vi "FileExplorer.vi"(0 "FolderPath":path, 1 "Copy Button":bool, 2 "Expand/Collapse":bool, 5 "Tree":string[](tree), 7 "SearchBar":string, 11 "error in (no error)":errorcluster) -> (4 "Report":string, 15 "error out":errorcluster)   [LabVIEW 2021]
doc: "This Vi acts as a file explorer. It populates the subfolders and files present in the selected folder path in tree along with the data of Last Modified,Type and Size of files."
uses:
  Controls/Operations.ctl
  Controls/Data Cluster.ctl
  Controls/State.ctl
panel:
  # "Instructions:\n\n-> Select the folder path to populate the subfolders and files present in tree.\n-> A report is generated for the folders whose checkbox is selected in tree.\n-> Press Collapse All button to collapse all nodes in tree and Expand All to expand\n      all nodes in tree.\n->  Enter a folder name in search bar and click enter to expand the nodes of searched folder.\n-> Click column headers such as Last Modified to sort the column itemns in ascending \n      and descending order.\n-> Select file to copy and click Copy button which opens a dialog box to choose the\n      folder path where the files are copied."
  # "Instructions:\n\n-> Select the Folder Path to populate the subfolders and files present in it in tree.\n->  Can select multiple files of same folder and press Copy button to copy those files.\n->  Clicking a Copy button opens a dialog box to choose the destination folder path \n       where the files are copied.\n->  A report is generated for the folders whose checkbox is selected in tree.\n->  Press Collapse All button to collapse all nodes in tree and Expand all to expand \n       all nodes in tree.\n->   Enter a folder name in SearchBar and press Search to search for a particular folder\n       in tree.\n->   Press column headers such as Last Modified to sort the column items in ascending \n        or descending order."
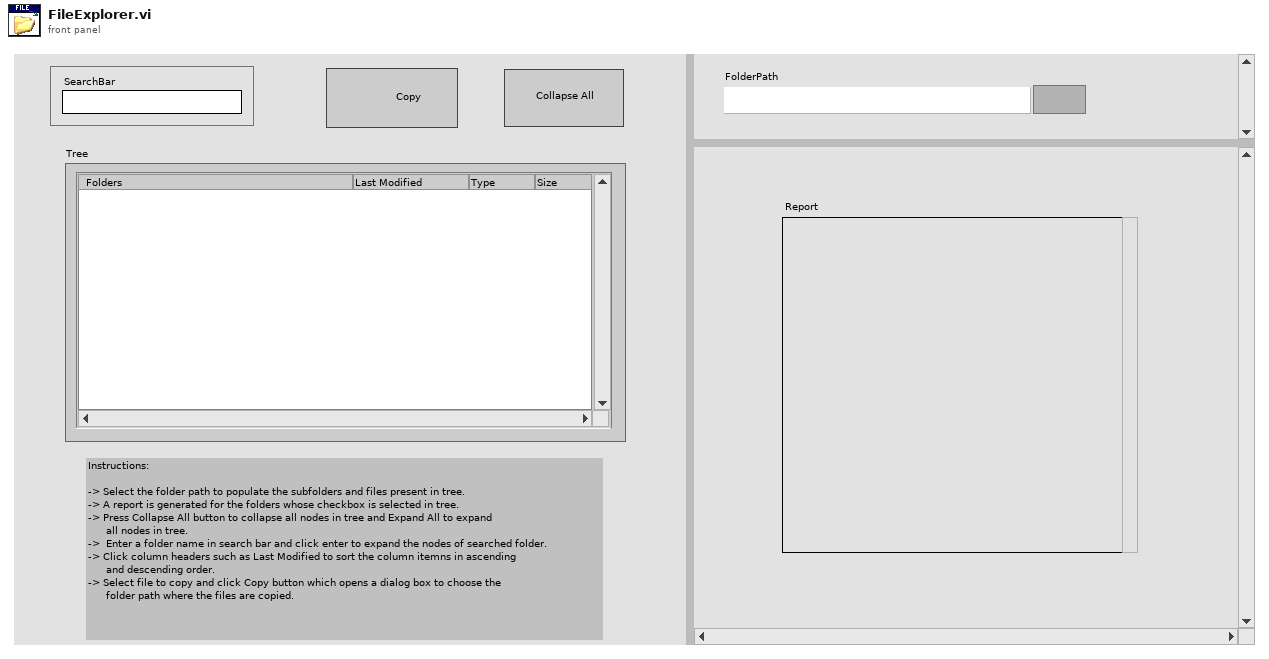
[diagram p1: front panel]
types:
  T1 = typedef "State.ctl" = cluster{"State":string, "Data":variant}
  T2 = typedef "Data Cluster.ctl" = cluster{"Stop user event":refnum<user-event>, "FolderPath":path, "FolderName":string, "FolderPathArray":path[], "FilePathArray":path[], "Index":i32, "No.of Folders":i32, "SelectedTags":string[], "SelectedFilePaths":path[], "SearchTag":string, "Column":i32, "Toggle":bool, "FolderTag":string, "ActiveTag":string, "ListBox":i32, "Report":string}
  T3 = typedef "Operations.ctl" = enum16{"Create", "Enqueue", "Enqueue N", "Enstack", "Dequeue", "Flush", "Release"}
  T4 = typedef "LVPoint32TypeDef.ctl" = cluster{"Horizontal":i32, "Vertical":i32}
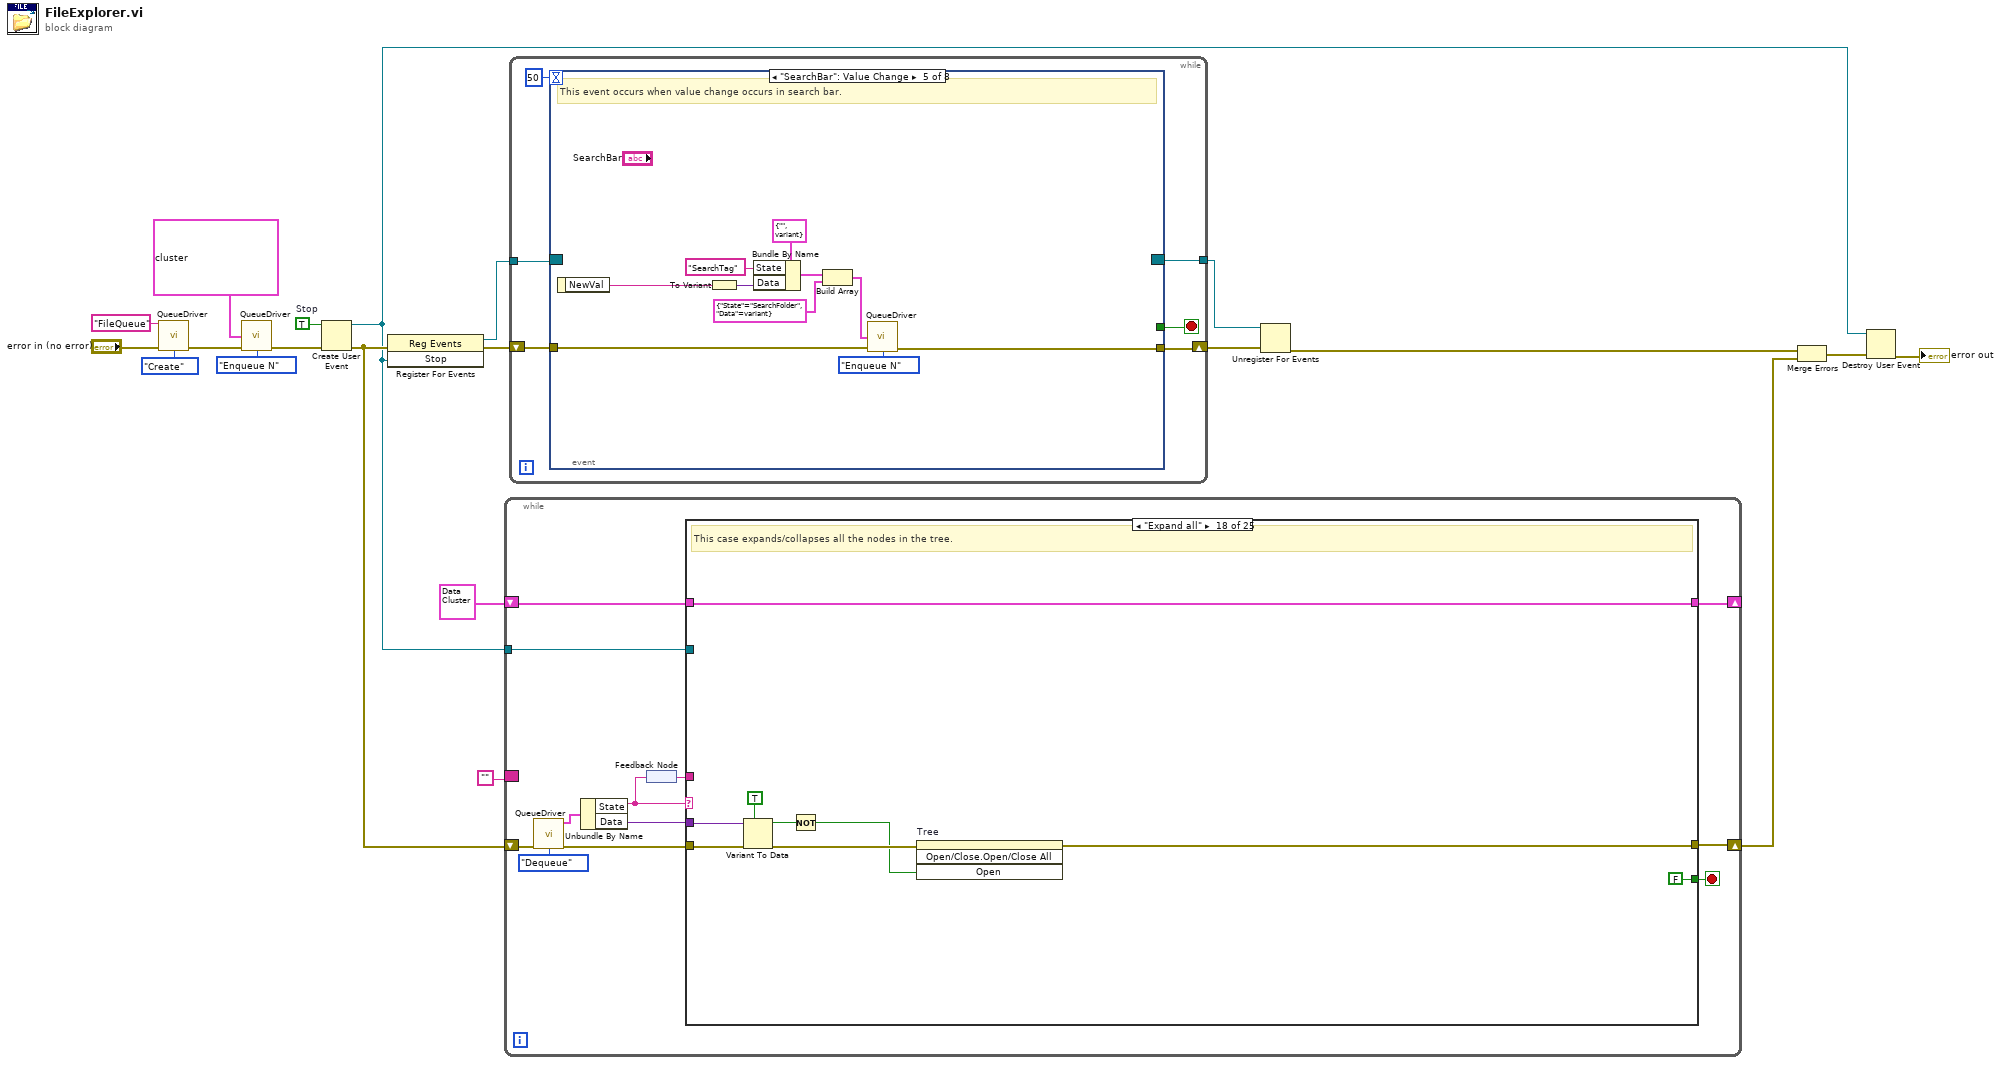
[diagram p0: block diagram]
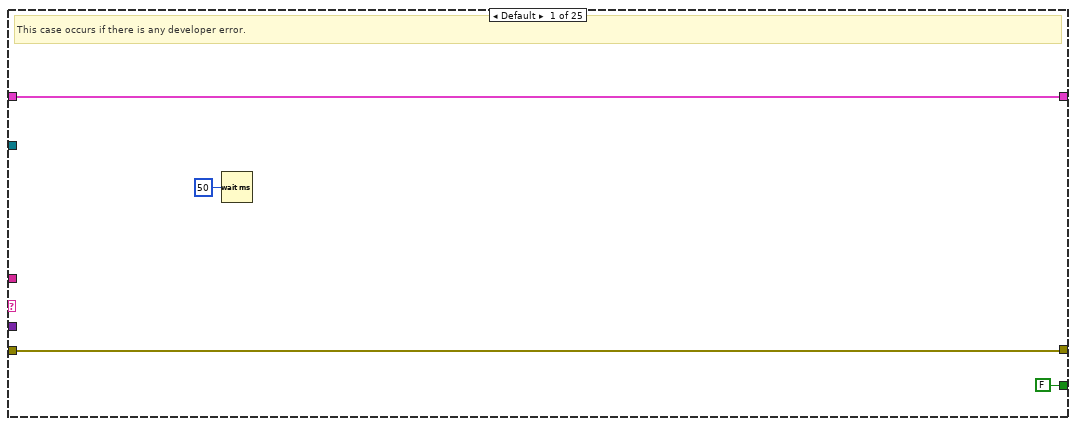
[diagram p2: hidden frame]
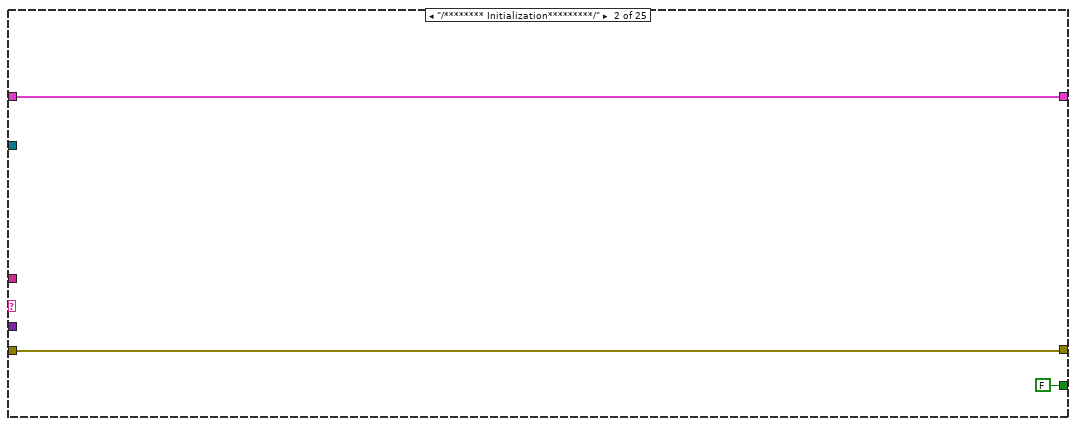
[diagram p3: hidden frame]
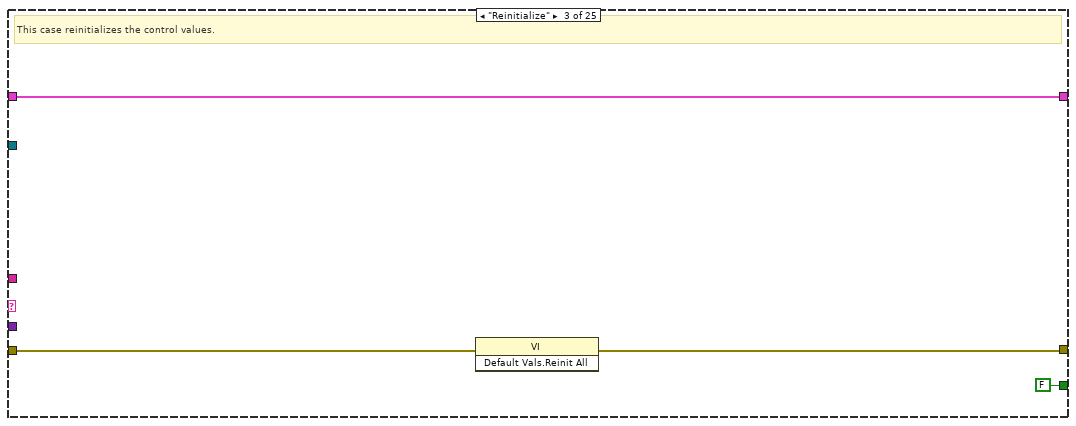
[diagram p4: hidden frame]
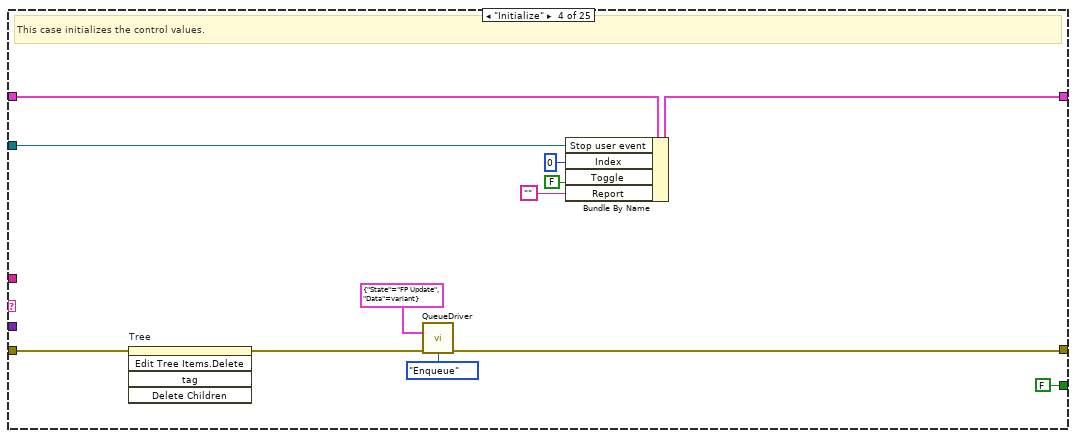
[diagram p5: hidden frame]
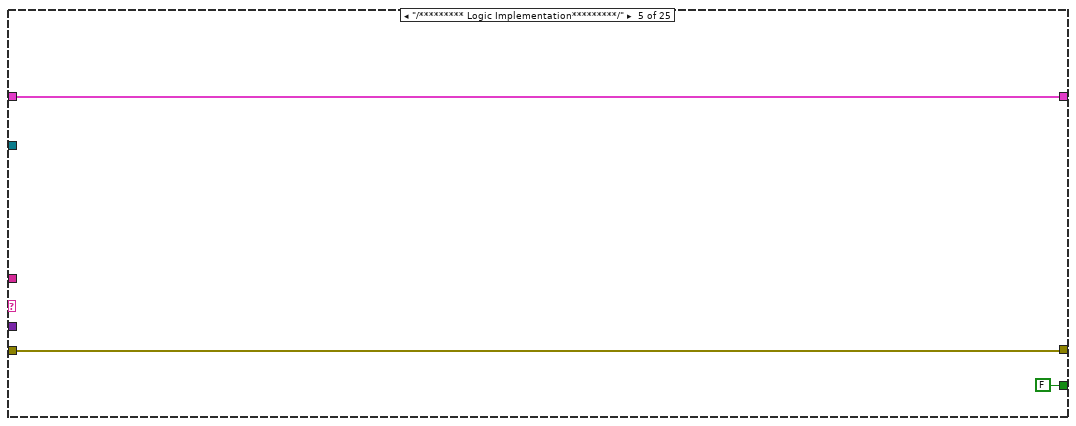
[diagram p6: hidden frame]
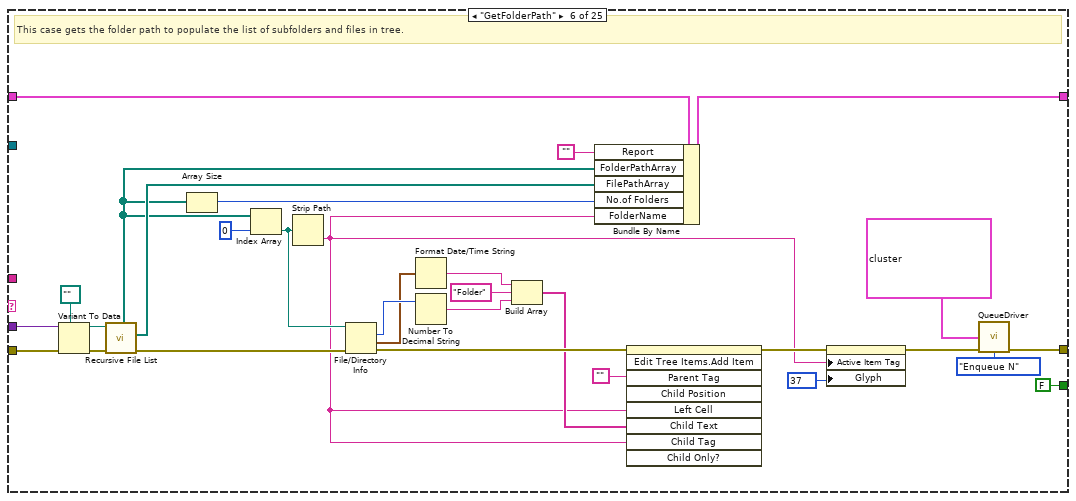
[diagram p7: hidden frame]
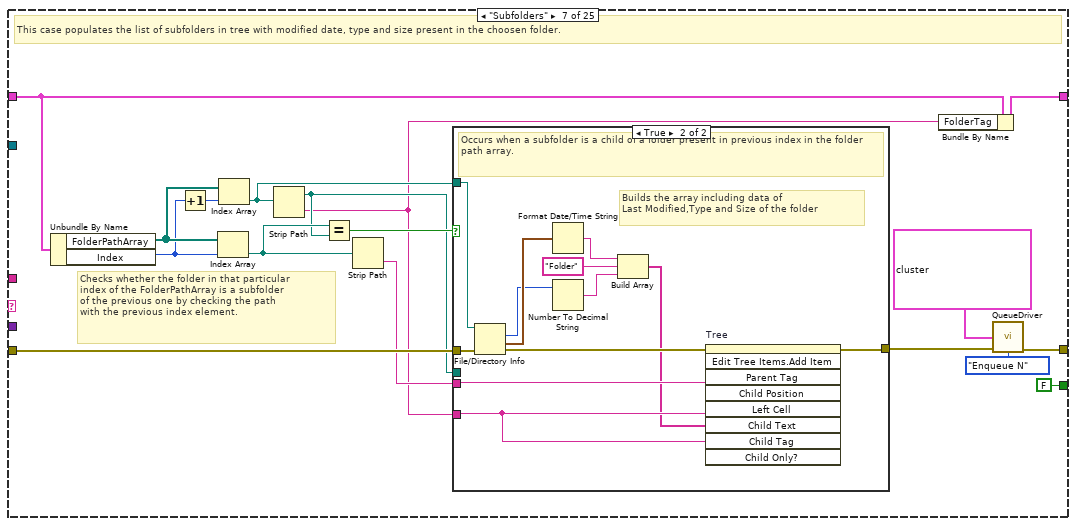
[diagram p8: hidden frame]
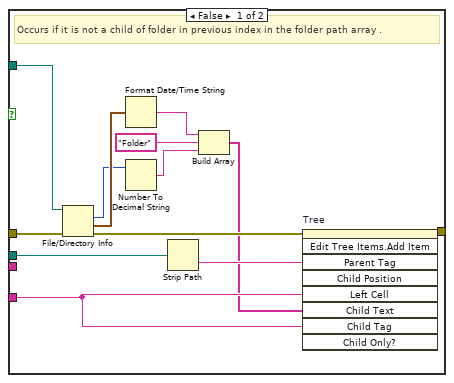
[diagram p9: hidden frame]
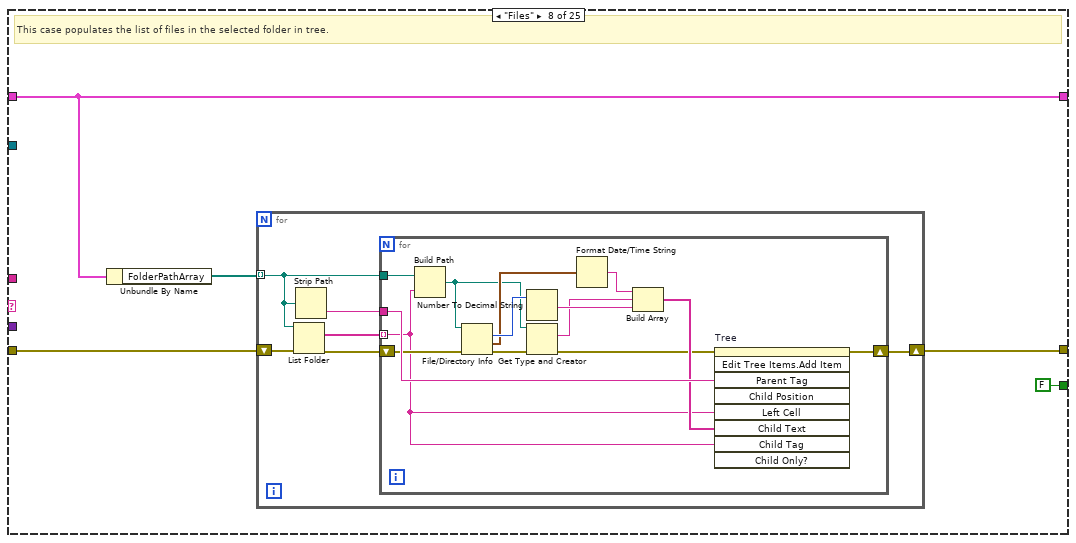
[diagram p10: hidden frame]
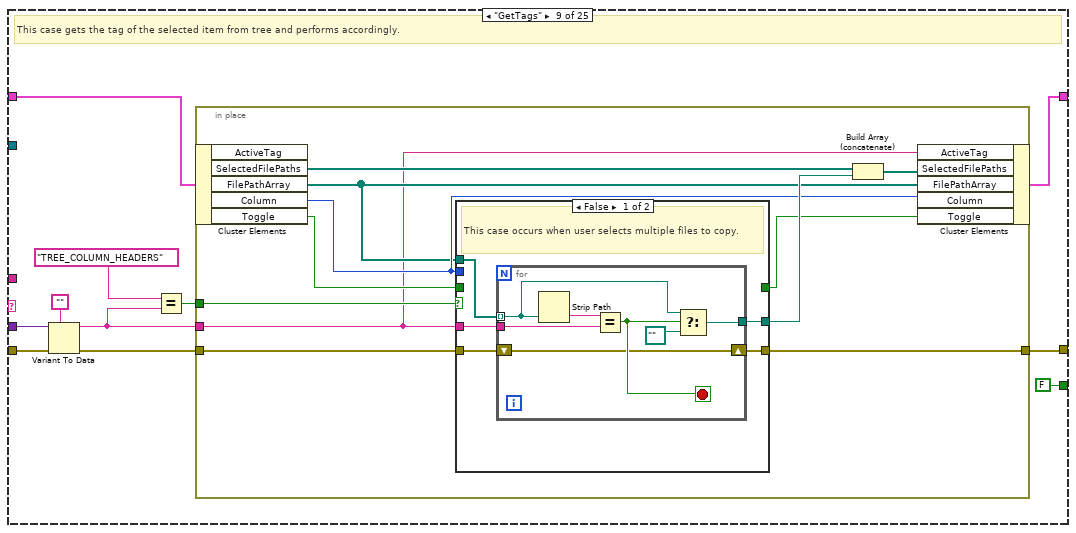
[diagram p11: hidden frame]
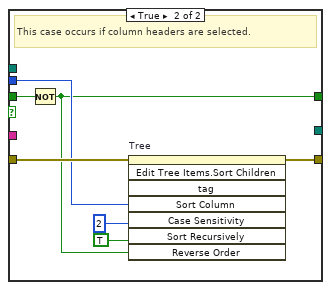
[diagram p12: hidden frame]
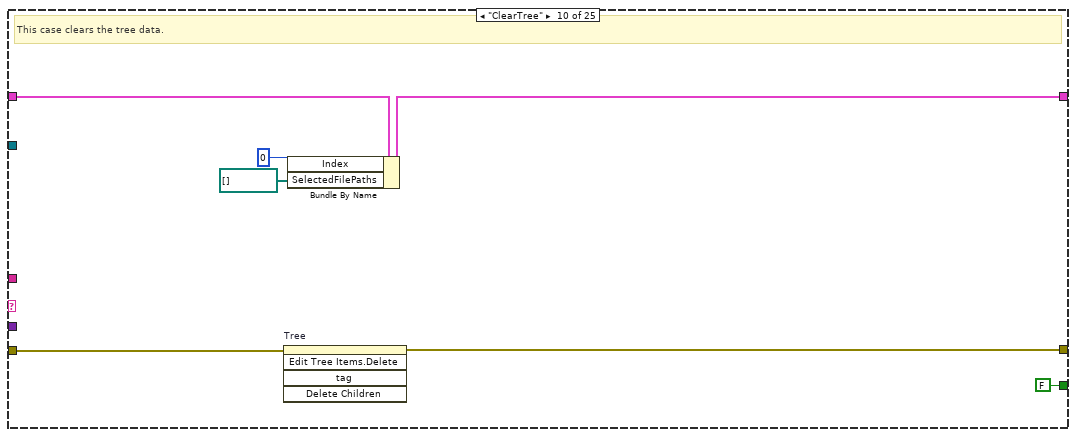
[diagram p13: hidden frame]
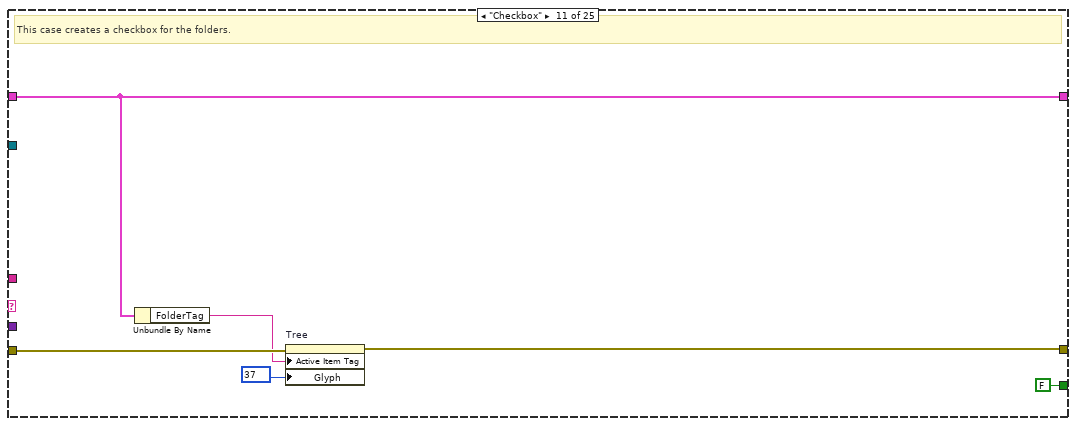
[diagram p14: hidden frame]
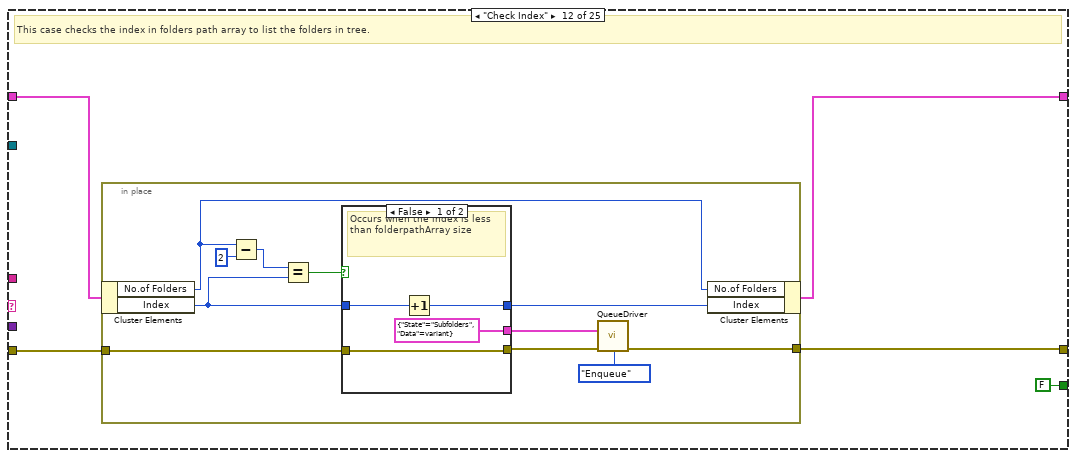
[diagram p15: hidden frame]
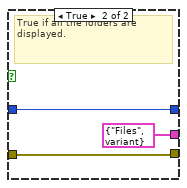
[diagram p16: hidden frame]
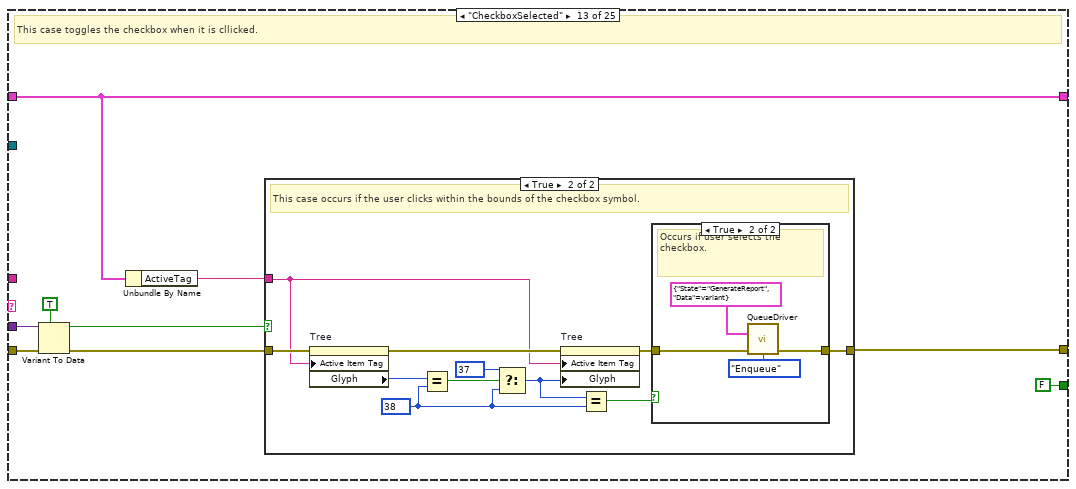
[diagram p17: hidden frame]
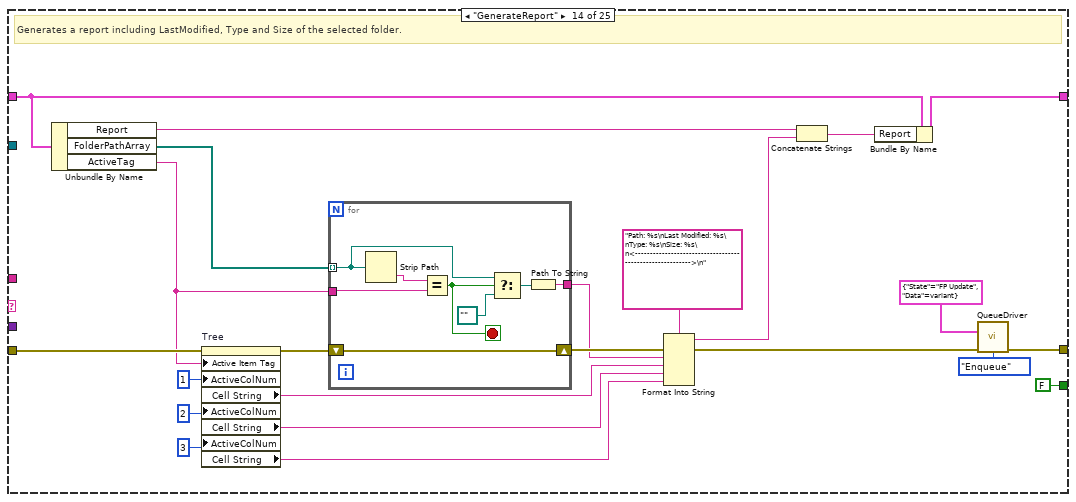
[diagram p20: hidden frame]
diagram:
  w20 = TRUE  # Stop
  n1 = call "QueueDriver.vi"("Queue Name"="FileQueue", "error in (no error)"="error in (no error)", "Operations"=Operations."Create") -> ("error out"=w15:errorcluster)  [unwired: 11 in, 1 out]
  n2 = call "QueueDriver.vi"("State[]"=T1[] [{"State"="Reinitialize", "Data"=variant}, {"State"="Initialize", "Data"=variant}], "error in (no error)"=w15, "Operations"=Operations."Enqueue N") -> ("error out"=w14:errorcluster)  [unwired: 11 in, 1 out]
  n3 = Create User Event(user event datatype=w20, error in=w14) -> (user event=w4:refnum<user-event>, error out=w17:errorcluster)
  n4 = register-events(error in=w17, w4) -> (reference out=w18:refnum<event-registration>, error out=w19:errorcluster)  [unwired: 1 in]
  n5 = while {
    shift-right: [w29] -> w6
    shift-left: w17 -> [w27]
    border: "" ("Empty String Constant") -> [_]
    tunnel: w4 -> [w23]
    shift-right: [w21] -> _
    shift-left: T2 {"Stop user event"=refnum, "FolderPath"=path "", "FolderName"="", "FolderPathArray"=[], "FilePathArray"=[], "Index"=0, "No.of Folders"=0, "SelectedTags"=[], "SelectedFilePaths"=[], "SearchTag"="", "Column"=0, "Toggle"=FALSE, "FolderTag"="", "ActiveTag"="", "ListBox"=0, "Report"=""} -> [w22]
    stop <- w28 stop-if-true
    n6 = call "QueueDriver.vi"("error in (no error)"=w27, "Operations"=Operations."Dequeue") -> ("Dequeued Element"=w25:T1, "error out"=w26:errorcluster)  [unwired: 12 in]
    n7 = Unbundle By Name(w25) -> ("State"=w32:string, "Data"=w30:variant)
    n8 = feedback-in #1(w32) -> ()
    n9 = feedback #1() -> (w31:string)
    n10 = case shown="\"Expand all\"" w32 {
      tunnel: w26 -> [w36 w39 w43 w52 w58 w88 w102 w134 w166 w202 w208 w214 w241 w281 w297 w303 w316 w337 w345 w348 w352 w355 w361 w381 w386]
      tunnel: w31 -> [_ _ _ _ _ _ _ _ _ _ _ _ _ _ _ _ _ _ _ _ _ _ w360 _ _]
      tunnel: w30 -> [_ _ _ _ _ w87 _ _ w165 _ _ _ w240 _ w296 _ _ w335 w343 _ _ _ _ _ _]
      tunnel: [w36 w39 w41 w46 w58 w79 w96 w132 w163 w203 w207 w213 w234 w262 w291 w299 w318 w332 w344 w348 w352 w355 w359 w381 w385] -> w29
      tunnel: [FALSE FALSE FALSE FALSE FALSE FALSE FALSE FALSE FALSE FALSE FALSE FALSE FALSE FALSE FALSE FALSE FALSE FALSE FALSE FALSE FALSE FALSE FALSE FALSE TRUE] -> w28
      tunnel: w23 -> [_ _ _ w54 _ _ _ _ _ _ _ _ _ _ _ _ _ _ _ _ _ _ _ _ _]
      tunnel: w22 -> [w35 w38 w42 w55 w57 w83 w92 w135 w158 w201 w209 w211 w238 w266 w294 w302 w313 w336 w341 w347 w351 w354 w358 w380 w382]
      tunnel: [w35 w38 w42 w53 w57 w82 w91 w135 w157 w200 w209 w210 w238 w265 w293 w302 w312 w336 w339 w347 w351 w354 w358 w380 w382] -> w21
      frame Default {
        # "This case occurs if there is any developer error."
        n11 = Wait (ms)(milliseconds to wait=u32 50) -> ()  [unwired: 1 out]
      }
      frame "/******** Initialization*********/" {
      }
      frame "Reinitialize" {
        # "This case reinitializes the control values."
        n12 = invoke on="Invoke Node" class="VI" method="Default Vals.Reinit All"(error in=w43) -> (error out=w41:errorcluster)  [unwired: 2 in, 2 out]
      }
      frame "Initialize" {
        # "This case initializes the control values."
        n13 = invoke on="Tree" class="Tree (strict)" method="Edit Tree Items.Delete"(error in=w52) -> (error out=w49:errorcluster)  [unwired: 4 in, 4 out]
        n14 = call "QueueDriver.vi"("State"=T1 {"State"="FP Update", "Data"=variant}, "error in (no error)"=w49, "Operations"=Operations."Enqueue") -> ("error out"=w46:errorcluster)  [unwired: 11 in, 1 out]
        n15 = Bundle By Name(cluster=w55, "Stop user event"=w54, "Index"=0, "Toggle"=FALSE, "Report"="" ("Empty String Constant")) -> (w53:T2)
      }
      frame "/********* Logic Implementation*********/" {
      }
      frame "GetFolderPath" {
        # "This case gets the folder path to populate the list of subfolders and files in tree."
        n16 = Variant To Data(error in=w88, type=path "" ("NewVal"), Variant=w87) -> (data=w84:path, error out=w85:errorcluster)
        n17 = call <vilib>:"Recursive File List.vi"("error in (no error)"=w85, "Folder Path"=w84) -> ("error out"=w72:errorcluster, "All Files in Dir"=w81:path[], "All Folders"=w77:path[])  [unwired: 5 in, 2 out]
        n18 = Array Size(array=w77) -> (size(s)=w76:i32)
        n19 = Index Array(array=w77, index=0) -> (element=w68:path)
        n20 = Strip Path(path=w68) -> (name=w64:string)  [unwired: 1 out]
        n21 = File/Directory Info(path=w68, error in=w72) -> (size=w73:i64, last mod=w70:timestamp, error out=w71:errorcluster)  [unwired: 4 out]
        n22 = Format Date/Time String(seconds (now)=w70) -> (date/time string=w69:string)  [unwired: 2 in]
        n23 = Number To Decimal String(number=w73) -> (decimal integer string=w74:string)  [unwired: 1 in]
        n24 = Build Array(w69, "Folder" ("element"), w74) -> (w67:string[])
        n25 = Bundle By Name(cluster=w83, "Report"="" ("Empty String Constant"), "FolderPathArray"=w77, "FilePathArray"=w81, "No.of Folders"=w76, "FolderName"=w64) -> (w82:T2)
        n26 = invoke on="Tree" class="Tree (strict)" method="Edit Tree Items.Add Item"(error in=w71, "Parent Tag"="" ("Empty String Constant"), "Left Cell"=w64, "Child Text"=w67, "Child Tag"=w64) -> (error out=w66:errorcluster)  [unwired: 4 in, 8 out]
        n27 = property on="Tree" class="Tree (strict)"(error in=w66, "Active Item Tag"=w64, "Glyph"=37) -> (error out=w65:errorcluster)  [unwired: 1 in, 1 out]
        n28 = call "QueueDriver.vi"("State[]"=T1[] [{"State"="FP Update", "Data"=variant}, {"State"="Subfolders", "Data"=variant}], "error in (no error)"=w65, "Operations"=Operations."Enqueue N") -> ("error out"=w79:errorcluster)  [unwired: 11 in, 1 out]
      }
      frame "Subfolders" {
        # "Checks whether the folder in that particular\nindex of the FolderPathArray is a subfolder \nof the previous one by checking the path\nwith the previous index element."
        # "This case populates the list of subfolders in tree with modified date, type and size present in the choosen folder."
        n29 = Unbundle By Name(w92) -> ("FolderPathArray"=w105:path[], "Index"=w104:i32)
        n30 = Increment(x=w104) -> (x+1=w103:i32)
        n31 = Index Array(array=w105, index=w104) -> (element=w100:path)
        n32 = Index Array(array=w105, index=w103) -> (element=w94:path)
        n33 = Strip Path(path=w94) -> (stripped path=w98:path, name=w90:string)
        n34 = Equal?(x=w100, y=w98) -> (x = y?=w101:bool)
        n35 = Strip Path(path=w100) -> (name=w99:string)  [unwired: 1 out]
        n36 = case shown="True" w101 {
          tunnel: w102 -> [w112 w124]
          tunnel: [w118 w130] -> w97
          tunnel: w99 -> [_ w129]
          tunnel: w90 -> [w117 w128]
          tunnel: w98 -> [w107 _]
          tunnel: w94 -> [w106 w125]
          frame False {
            # "Occurs if it is not a child of folder in previous index in the folder path array ."
            n37 = File/Directory Info(path=w106, error in=w112) -> (size=w109:i64, last mod=w110:timestamp, error out=w111:errorcluster)  [unwired: 4 out]
            n38 = Format Date/Time String(seconds (now)=w110) -> (date/time string=w115:string)  [unwired: 2 in]
            n39 = Number To Decimal String(number=w109) -> (decimal integer string=w113:string)  [unwired: 1 in]
            n40 = Strip Path(path=w107) -> (name=w116:string)  [unwired: 1 out]
            n41 = Build Array(w115, "Folder" ("element"), w113) -> (w108:string[])
            n42 = invoke on="Tree" class="Tree (strict)" method="Edit Tree Items.Add Item"(error in=w111, "Parent Tag"=w116, "Left Cell"=w117, "Child Text"=w108, "Child Tag"=w117) -> (error out=w118:errorcluster)  [unwired: 4 in, 8 out]
          }
          frame True {
            # "Builds the array including data of\nLast Modified,Type and Size of the folder"
            # "Occurs when a subfolder is a child of a folder present in previous index in the folder path array."
            n43 = File/Directory Info(path=w125, error in=w124) -> (size=w126:i64, last mod=w127:timestamp, error out=w123:errorcluster)  [unwired: 4 out]
            n44 = Format Date/Time String(seconds (now)=w127) -> (date/time string=w122:string)  [unwired: 2 in]
            n45 = Number To Decimal String(number=w126) -> (decimal integer string=w120:string)  [unwired: 1 in]
            n46 = Build Array(w122, "Folder" ("element"), w120) -> (w119:string[])
            n47 = invoke on="Tree" class="Tree (strict)" method="Edit Tree Items.Add Item"(error in=w123, "Parent Tag"=w129, "Left Cell"=w128, "Child Text"=w119, "Child Tag"=w128) -> (error out=w130:errorcluster)  [unwired: 4 in, 8 out]
          }
        }
        n48 = Bundle By Name(cluster=w92, "FolderTag"=w90) -> (w91:T2)
        n49 = call "QueueDriver.vi"("State[]"=T1[] [{"State"="Checkbox", "Data"=variant}, {"State"="Check Index", "Data"=variant}], "error in (no error)"=w97, "Operations"=Operations."Enqueue N") -> ("error out"=w96:errorcluster)  [unwired: 11 in, 1 out]
      }
      frame "Files" {
        # "This case populates the list of files in the selected folder in tree."
        n50 = Unbundle By Name(w135) -> ("FolderPathArray"=w133:path[])
        n51 = for {
          shift-right: [w141] -> w132
          shift-left: w134 -> [w139]
          tunnel: w133 -> [w136] mode=indexing
          n52 = List Folder(path=w136, error in=w139) -> (filenames=w137:string[], error out=w138:errorcluster)  [unwired: 2 in, 2 out]
          n53 = Strip Path(path=w136) -> (name=w140:string)  [unwired: 1 out]
          n54 = for {
            shift-right: [w155] -> w141
            shift-left: w138 -> [w153]
            tunnel: w140 -> [w154]
            tunnel: w137 -> [w145] mode=indexing
            tunnel: w136 -> [w146]
            n55 = Build Path(base path=w146, name or relative path=w145) -> (appended path=w144:path)
            n56 = File/Directory Info(path=w144, error in=w153) -> (size=w152:i64, last mod=w149:timestamp, error out=w143:errorcluster)  [unwired: 4 out]
            n57 = Number To Decimal String(number=w152) -> (decimal integer string=w151:string)  [unwired: 1 in]
            n58 = Get Type and Creator(4:w143, 7:w144) -> (0:w142:errorcluster, 2:w150:string)  [unwired: 2 out]
            n59 = Format Date/Time String(seconds (now)=w149) -> (date/time string=w148:string)  [unwired: 2 in]
            n60 = Build Array(w148, w150, w151) -> (w147:string[])
            n61 = invoke on="Tree" class="Tree (strict)" method="Edit Tree Items.Add Item"(error in=w142, "Parent Tag"=w154, "Left Cell"=w145, "Child Text"=w147, "Child Tag"=w145) -> (error out=w155:errorcluster)  [unwired: 4 in, 8 out]
          }
        }
      }
      frame "GetTags" {
        # "This case gets the tag of the selected item from tree and performs accordingly."
        n62 = Variant To Data(error in=w166, type="" ("Empty String Constant"), Variant=w165) -> (data=w160:string, error out=w164:errorcluster)
        n63 = Equal?(x="TREE_COLUMN_HEADERS", y=w160) -> (x = y?=w161:bool)
        n64 = in-place "In Place Element Structure" {
          in-place-border: w164 -> [w177]
          in-place-border: [w175] -> w163
          in-place-border: w161 -> [w174]
          in-place-border: w160 -> [w167]
          n65 = in-place-cluster #2(w158) -> ("SelectedFilePaths"=w173:path[], "FilePathArray"=w168:path[], "Column"=w169:i32, "Toggle"=w172:bool)  [unwired: 1 out]
          n66 = case shown="False" w174 {
            tunnel: w177 -> [w182 w196]
            tunnel: w168 -> [w181 _]
            tunnel: [w180 _] -> w176
            tunnel: [w179 w195] -> w175
            tunnel: w167 -> [w178 _]
            tunnel: w169 -> [_ w194]
            tunnel: w172 -> [_ w191]
            tunnel: [_ w190] -> w171
            frame False {
              # "This case occurs when user selects multiple files to copy."
              n67 = for {
                tunnel: w181 -> [w186] mode=indexing
                tunnel: w178 -> [w188]
                tunnel: [w184] -> w180
                shift-right: [w183] -> w179
                shift-left: w182 -> [w183]
                stop <- w187 stop-if-true
                n68 = Strip Path(path=w186) -> (name=w189:string)  [unwired: 1 out]
                n69 = Equal?(x=w189, y=w188) -> (x = y?=w187:bool)
                n70 = Select(t=w186, s=w187, f=path "") -> (s? t:f=w184:path)
              }
            }
            frame True {
              # "This case occurs if column headers are selected."
              n71 = Not(x=w191) -> (.not. x?=w190:bool)
              n72 = invoke on="Tree" class="Tree (strict)" method="Edit Tree Items.Sort Children"(error in=w196, "Sort Column"=w194, "Case Sensitivity"=2, "Sort Recursively"=TRUE ("Sort Recursively?"), "Reverse Order"=w190) -> (error out=w195:errorcluster)  [unwired: 3 in, 7 out]
            }
          }
          n73 = Build Array (concatenate)(w173, w176) -> (w170:path[])
          n74 = in-place-cluster #2("ActiveTag"=w167, "SelectedFilePaths"=w170, "FilePathArray"=w168, "Column"=w169, "Toggle"=w171) -> (w157:T2)
        }
      }
      frame "ClearTree" {
        # "This case clears the tree data."
        n75 = invoke on="Tree" class="Tree (strict)" method="Edit Tree Items.Delete"(error in=w202) -> (error out=w203:errorcluster)  [unwired: 4 in, 4 out]
        n76 = Bundle By Name(cluster=w201, "Index"=0, "SelectedFilePaths"=path[] []) -> (w200:T2)
      }
      frame "Checkbox" {
        # "This case creates a checkbox for the folders."
        n77 = Unbundle By Name(w209) -> ("FolderTag"=w206:string)
        n78 = property on="Tree" class="Tree (strict)"(error in=w208, "Active Item Tag"=w206, "Glyph"=37) -> (error out=w207:errorcluster)  [unwired: 1 in, 1 out]
      }
      frame "Check Index" {
        # "This case checks the index in folders path array to list the folders in tree."
        n79 = in-place "In Place Element Structure" {
          in-place-border: w214 -> [w223]
          in-place-border: [w218] -> w213
          n80 = in-place-cluster #3(w211) -> ("No.of Folders"=w215:i32, "Index"=w217:i32)
          n81 = Subtract(x=w215, y=2) -> (x-y=w224:i32)
          n82 = Equal?(x=w224, y=w217) -> (x = y?=w222:bool)
          n83 = case shown="False" w222 {
            tunnel: w223 -> [w228 w232]
            tunnel: [w228 w232] -> w221
            tunnel: [T1 {"State"="Subfolders", "Data"=variant} ("State") T1 {"State"="Files", "Data"=variant} ("State")] -> w219
            tunnel: w217 -> [w227 w230]
            tunnel: [w226 w230] -> w216
            frame False {
              # "Occurs when the index is less than folderpathArray size"
              n84 = Increment(x=w227) -> (x+1=w226:i32)
            }
            frame True {
              # "True if all the folders are displayed."
            }
          }
          n85 = call "QueueDriver.vi"("State"=w219, "error in (no error)"=w221, "Operations"=Operations."Enqueue") -> ("error out"=w218:errorcluster)  [unwired: 11 in, 1 out]
          n86 = in-place-cluster #3("No.of Folders"=w215, "Index"=w216) -> (w210:T2)
        }
      }
      frame "CheckboxSelected" {
        # "This case toggles the checkbox when it is cllicked."
        n87 = Variant To Data(error in=w241, type=TRUE, Variant=w240) -> (data=w237:bool, error out=w235:errorcluster)
        n88 = Unbundle By Name(w238) -> ("ActiveTag"=w236:string)
        n89 = case shown="True" w237 {
          tunnel: w236 -> [_ w248]
          tunnel: w235 -> [w242 w253]
          tunnel: [w242 w243] -> w234
          frame False {
            # "This case occurs if it is not within the bounds of the symbol."
          }
          frame True {
            w246 = 38
            # "This case occurs if the user clicks within the bounds of the checkbox symbol."
            n90 = property on="Tree" class="Tree (strict)"(error in=w253, "Active Item Tag"=w248) -> (error out=w249:errorcluster, "Glyph"=w252:i32)  [unwired: 1 in, 1 out]
            n91 = Equal?(x=w252, y=w246) -> (x = y?=w251:bool)
            n92 = Select(t=37, s=w251, f=w246) -> (s? t:f=w247:i32)
            n93 = property on="Tree" class="Tree (strict)"(error in=w249, "Active Item Tag"=w248, "Glyph"=w247) -> (error out=w245:errorcluster)  [unwired: 1 in, 1 out]
            n94 = Equal?(x=w247, y=w246) -> (x = y?=w244:bool)
            n95 = case shown="True" w244 {
              tunnel: w245 -> [w254 w258]
              tunnel: [w254 w257] -> w243
              frame False {
                # "Occurs if it is unchecked."
              }
              frame True {
                # "Occurs if user selects the checkbox."
                n96 = call "QueueDriver.vi"("State"=T1 {"State"="GenerateReport", "Data"=variant}, "error in (no error)"=w258, "Operations"=Operations."Enqueue") -> ("error out"=w257:errorcluster)  [unwired: 11 in, 1 out]
              }
            }
          }
        }
      }
      frame "GenerateReport" {
        # "Generates a report including LastModified, Type and Size of the selected folder."
        n97 = Unbundle By Name(w266) -> ("Report"=w268:string, "FolderPathArray"=w277:path[], "ActiveTag"=w276:string)
        n98 = property on="Tree" class="Tree (strict)"(error in=w281, "Active Item Tag"=w276, "ActiveColNum"=1 ("Active Cell:Active Column Number"), "ActiveColNum"=2 ("Active Cell:Active Column Number"), "ActiveColNum"=3 ("Active Cell:Active Column Number")) -> (error out=w275:errorcluster, "Cell String"=w271:string, "Cell String"=w270:string, "Cell String"=w269:string)  [unwired: 1 in, 1 out]
        n99 = for {
          tunnel: w277 -> [w282] mode=indexing
          tunnel: w276 -> [w288]
          tunnel: [w287] -> w272
          shift-right: [w286] -> w274
          shift-left: w275 -> [w286]
          stop <- w283 stop-if-true
          n100 = Strip Path(path=w282) -> (name=w289:string)  [unwired: 1 out]
          n101 = Equal?(x=w289, y=w288) -> (x = y?=w283:bool)
          n102 = Select(t=w282, s=w283, f=path "") -> (s? t:f=w285:path)
          n103 = Path To String(path=w285) -> (string=w287:string)
        }
        n104 = Format Into String(format string="Path: %s\nLast Modified: %s\nType: %s\nSize: %s\n<--------------------------------------------------------->\n", error in=w274, w272, w271, w270, w269) -> (resulting string=w267:string, error out=w263:errorcluster)  [unwired: 1 in]
        n105 = Concatenate Strings(w268, w267) -> (w264:string)
        n106 = Bundle By Name(cluster=w266, "Report"=w264) -> (w265:T2)
        n107 = call "QueueDriver.vi"("State"=T1 {"State"="FP Update", "Data"=variant}, "error in (no error)"=w263, "Operations"=Operations."Enqueue") -> ("error out"=w262:errorcluster)  [unwired: 11 in, 1 out]
      }
      frame "SearchTag" {
        # "This case gets the folder name that user enters in SearchBar."
        n108 = Variant To Data(error in=w297, type="" ("Empty String Constant"), Variant=w296) -> (data=w292:string, error out=w291:errorcluster)
        n109 = Bundle By Name(cluster=w294, "SearchTag"=w292) -> (w293:T2)
      }
      frame "SearchFolder" {
        # "This case expands the contents of the searched folder."
        n110 = Unbundle By Name(w302) -> ("SearchTag"=w300:string)
        n111 = Empty String/Path?(string/path=w300) -> (empty?=w301:bool)
        n112 = case shown="False" w301 {
          tunnel: w303 -> [w308 w309]
          tunnel: w300 -> [w305 _]
          tunnel: [w306 w309] -> w299
          frame False {
            # "Occurs if the string is not empty."
            n113 = invoke on="Tree" class="Tree (strict)" method="Open/Close.Ensure Visible"(error in=w308, "tag"=w305) -> (error out=w307:errorcluster)  [unwired: 2 in, 3 out]
            n114 = invoke on="Tree" class="Tree (strict)" method="Open/Close.Item"(error in=w307, "tag"=w305, "Open"=TRUE ("Open?")) -> (error out=w306:errorcluster)  [unwired: 2 in, 4 out]
          }
          frame True {
            # "Occurs if string is empty."
          }
        }
      }
      frame "CopyFiles" {
        # "This case copies the selected files into the destination location."
        n115 = call "File Dialog"("error in"=w316) -> ("selected path"=w314:path, "error out"=w315:errorcluster)  [unwired: 11 in, 2 out]
        n116 = Unbundle By Name(w313) -> ("SelectedFilePaths"=w317:path[])
        n117 = for {
          shift-right: [w322] -> w318
          shift-left: w315 -> [w323]
          tunnel: w317 -> [w319] mode=indexing
          tunnel: w314 -> [w321]
          n118 = Empty String/Path?(string/path=w319) -> (empty?=w320:bool)
          n119 = case shown="False" w320 {
            tunnel: w323 -> [w327 w328]
            tunnel: [w326 w328] -> w322
            tunnel: w321 -> [w325 _]
            tunnel: w319 -> [w324 _]
            frame False {
              # "Copies if path is not empty."
              n120 = Copy(8:w327, 10:w325, 11:w324) -> (0:w326:errorcluster)  [unwired: 2 in, 2 out]
            }
            frame True {
              # "Occurs if path is empty."
            }
          }
        }
        n121 = Bundle By Name(cluster=w313, "SelectedFilePaths"=path[] []) -> (w312:T2)
      }
      frame "Expand all" {
        # "This case expands/collapses all the nodes in the tree."
        n122 = Variant To Data(error in=w337, type=TRUE, Variant=w335) -> (data=w331:bool, error out=w333:errorcluster)
        n123 = Not(x=w331) -> (.not. x?=w330:bool)
        n124 = invoke on="Tree" class="Tree (strict)" method="Open/Close.Open/Close All"(error in=w333, "Open"=w330) -> (error out=w332:errorcluster)  [unwired: 2 in, 3 out]
      }
      frame "Column" {
        # "This case gets the the column number of selected item in tree."
        n125 = Variant To Data(error in=w345, type=0 ("Column"), Variant=w343) -> (data=w340:i32, error out=w344:errorcluster)
        n126 = Bundle By Name(cluster=w341, "Column"=w340) -> (w339:T2)
      }
      frame "/******** Front Panel Updates ********/" {
      }
      frame "FP Update" {
        # "This case updates the front panel indicators."
        n127 = Unbundle By Name(w351) -> ("Report"=→"Report":string)
      }
      frame "/********* Error Handling ********/" {
      }
      frame "Error" {
        # "This case handles the error if any occured."
        n128 = Unbundle By Name(w361) -> ("code"=w368:i32, "source"=w367:string)
        n129 = call <vilib>:"Clear Errors.vi"("error in (no error)"=w361) -> ("error out"=w370:errorcluster)  [unwired: 5 in, 1 out]
        n130 = Format Into String(format string="Error occurred in state \"%s\"!!\nError Code: %d\nError Source: %s\n\nDo you wish to continue?", error in=w370, w360, w368, w367) -> (resulting string=w366:string, error out=w363:errorcluster)  [unwired: 1 in]
        n131 = Unbundle By Name(w358) -> ("Stop user event"=w357:refnum<user-event>)
        n132 = Two Button Dialog(message=w366, 1:"Exit" ("F button name (\"Cancel\")"), 2:"Continue" ("T button name (\"OK\")")) -> (T button?=w362:bool)
        n133 = case shown="False" w362 {
          tunnel: w363 -> [w377 w378]
          tunnel: [w374 w378] -> w359
          tunnel: w357 -> [w371 _]
          frame False {
            # "This case occurs when user selects exit."
            n134 = Generate User Event(user event=w371, event data cluster=TRUE ("event data"), error in=w377) -> (error out=w375:errorcluster)  [unwired: 1 in, 1 out]
            n135 = call "QueueDriver.vi"("State"=T1 {"State"="Exit", "Data"=variant}, "error in (no error)"=w375, "Operations"=Operations."Enqueue") -> ("error out"=w374:errorcluster)  [unwired: 11 in, 1 out]
          }
          frame True {
            # "This case occurs when user selects to continue."
          }
        }
      }
      frame "/******** Stopping the running Vi ********/" {
      }
      frame "Exit" {
        # "This case stops the running vi."
        n136 = call "QueueDriver.vi"("error in (no error)"=w386, "Operations"=Operations."Flush") -> ("error out"=w387:errorcluster)  [unwired: 12 in, 1 out]
        n137 = call "QueueDriver.vi"("error in (no error)"=w387, "Operations"=Operations."Release") -> ("error out"=w385:errorcluster)  [unwired: 12 in, 1 out]
      }
    }
  }
  n138 = while {
    shift-right: [w391] -> w8
    shift-left: w19 -> [w392]
    tunnel: w18 -> [w393]
    tunnel: [w389] -> w9
    stop <- w390 stop-if-true
    n139 = event shown="[4] \"SearchBar\": Value Change" {
      selector: w393 -> [_ _ _ _ _ _ _ _]
      dyn-events: [_ _ _ _ _ _ _ _] -> w389
      timeout: 50 -> [_ _ _ _ _ _ _ _]
      tunnel: w392 -> [w395 w399 w412 w432 w443 w451 w455 w457]
      tunnel: [w395 w398 w411 w430 w442 w450 w454 w457] -> w391
      tunnel: [_ w400 _ _ _ _ _ TRUE] -> w390
      event Timeout {
        # "This event occurs when no other event occurs."
        n140 = event-data() -> ()  [unwired: 1 in, 1 out]
      }
      event Panel Close? {
        w400 = TRUE
        # "This event occurs when panel close is pressed and stops the running vi."
        n141 = event-data() -> ()  [unwired: 1 in, 1 out]
        n142 = call "QueueDriver.vi"("State"=T1 {"State"="Exit", "Data"=variant}, "error in (no error)"=w399, "Operations"=Operations."Enqueue") -> ("error out"=w398:errorcluster)  [unwired: 11 in, 1 out]
        n143 = event-data ("Event Filter Node")("Discard?"=w400) -> ()  [unwired: 1 in, 1 out]
      }
      event "FolderPath": Value Change {
        # "This event occurs when path value change is done by the user."
        n144 = event-data() -> ("NewVal"=w408:path)  [unwired: 1 in]
        n145 = To Variant(anything=w408) -> (Variant=w407:variant)
        n146 = Bundle By Name(cluster=T1 {"State"="", "Data"=variant} ("State"), "State"="GetFolderPath", "Data"=w407) -> (w402:T1)
        n147 = Bundle By Name(cluster=T1 {"State"="", "Data"=variant} ("State"), "State"="ClearTree") -> (w403:T1)
        n148 = Build Array(w403, w402) -> (w401:T1[])
        n149 = call "QueueDriver.vi"("State[]"=w401, "error in (no error)"=w412, "Operations"=Operations."Enqueue N") -> ("error out"=w411:errorcluster)  [unwired: 11 in, 1 out]
      }
      event "Tree": Mouse Down {
        # "This event occurs when a user selects an item in the tree."
        n150 = event-data() -> ("Coords"=w433:T4)  [unwired: 1 in]
        n151 = invoke on="Tree" class="Tree (strict)" method="Point To Row Column"(error in=w432, "Point"=w433) -> (error out=w431:errorcluster, "Tag"=w427:string, "Col"=w421:i32, "InGlyph"=w415:bool)  [unwired: 6 in, 4 out]
        n152 = To Variant(anything=w421) -> (Variant=w423:variant)
        n153 = To Variant(anything=w427) -> (Variant=w426:variant)
        n154 = To Variant(anything=w415) -> (Variant=w414:variant)
        n155 = Bundle By Name(cluster=T1 {"State"="", "Data"=variant} ("State"), "State"="Column", "Data"=w423) -> (w420:T1)
        n156 = Bundle By Name(cluster=T1 {"State"="", "Data"=variant} ("State"), "State"="GetTags", "Data"=w426) -> (w419:T1)
        n157 = Bundle By Name(cluster=T1 {"State"="", "Data"=variant} ("State"), "State"="CheckboxSelected", "Data"=w414) -> (w413:T1)
        n158 = Build Array(w420, w419, w413) -> (w418:T1[])
        n159 = call "QueueDriver.vi"("State[]"=w418, "error in (no error)"=w431, "Operations"=Operations."Enqueue N") -> ("error out"=w430:errorcluster)  [unwired: 11 in, 1 out]
      }
      event "SearchBar": Value Change {
        # "This event occurs when value change occurs in search bar."
        n160 = event-data() -> ("NewVal"=w440:string)  [unwired: 1 in]
        n161 = To Variant(anything=w440) -> (Variant=w438:variant)
        n162 = Bundle By Name(cluster=T1 {"State"="", "Data"=variant} ("State"), "State"="SearchTag", "Data"=w438) -> (w436:T1)
        n163 = Build Array(w436, T1 {"State"="SearchFolder", "Data"=variant} ("State")) -> (w434:T1[])
        n164 = call "QueueDriver.vi"("State[]"=w434, "error in (no error)"=w443, "Operations"=Operations."Enqueue N") -> ("error out"=w442:errorcluster)  [unwired: 11 in, 1 out]
      }
      event "Expand/Collapse": Value Change {
        # "This event occurs when Expand/Collapse button is pressed."
        n165 = event-data() -> ("NewVal"=w448:bool)  [unwired: 1 in]
        n166 = To Variant(anything=w448) -> (Variant=w446:variant)
        n167 = Bundle By Name(cluster=T1 {"State"="", "Data"=variant} ("State"), "State"="Expand all", "Data"=w446) -> (w444:T1)
        n168 = call "QueueDriver.vi"("State"=w444, "error in (no error)"=w451, "Operations"=Operations."Enqueue") -> ("error out"=w450:errorcluster)  [unwired: 11 in, 1 out]
      }
      event "Copy Button": Value Change {
        # "This event occurs when Copy button is pressed."
        n169 = event-data() -> ()  [unwired: 1 in, 1 out]
        n170 = call "QueueDriver.vi"("State"=T1 {"State"="CopyFiles", "Data"=variant}, "error in (no error)"=w455, "Operations"=Operations."Enqueue") -> ("error out"=w454:errorcluster)  [unwired: 11 in, 1 out]
      }
      event User Event {
        # "This user event stops the runing vi."
        n171 = event-data() -> ()  [unwired: 1 in, 1 out]
      }
    }
  }
  n172 = Unregister For Events(event registration refnum=w9, error in=w8) -> (error out=w7:errorcluster)
  n173 = Merge Errors(w7, w6) -> (w5:errorcluster)
  n174 = Destroy User Event(user event=w4, error in=w5) -> (error out=→"error out":errorcluster)
